vi "Display Hours Minutes Seconds.vi"() -> ()   [LabVIEW 2012]
panel:
  out "Time to Match (Hours:Minutes:Seconds)":dbl format="%<%H:%M:%S>t"
  out "Time to Match (Seconds / Milliseconds)":dbl
  out "Time to Match":i32
  out "No of Interations":i32
  out "Current Number":i32
  in  "Number to Match":i32=500000 min=0 max=1000000 step=1 format="%.0g"
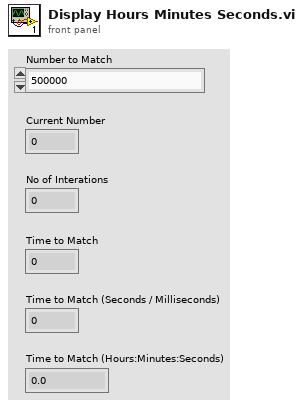
[diagram p1: front panel]
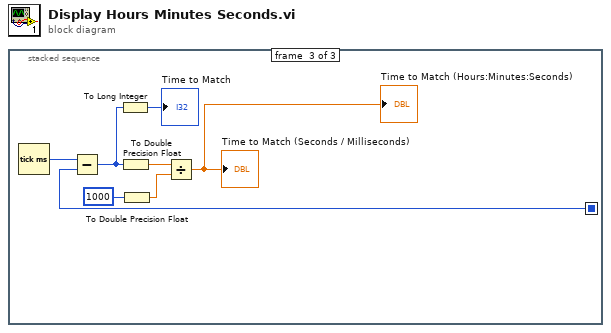
[diagram p0: block diagram]
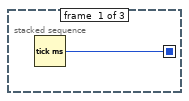
[diagram p2: hidden frame]
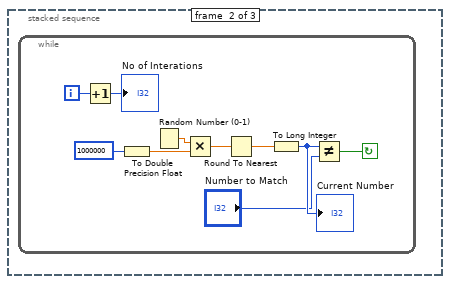
[diagram p3: hidden frame]
diagram:
  n1 = stacked-sequence {
    seq-local: [w1 _ _] -> [_ _ w18]
    frame #0 {
      n2 = Tick Count (ms)() -> (millisecond timer value=w1:u32)
    }
    frame #1 {
      n3 = while {
        i -> [w5]
        stop <- w2 continue-if-true
        n4 = Increment(x=w5) -> (x+1=→"No of Interations":i32)
        n5 = To Double Precision Float(number=1000000) -> (double precision float=w9:dbl)
        n6 = Random Number (0-1)() -> (number: 0 to 1=w11:dbl)
        n7 = Multiply(x=w11, y=w9) -> (x*y=w8:dbl)
        n8 = Round To Nearest(number=w8) -> (nearest integer value=w7:dbl)
        n9 = To Long Integer(number=w7) -> (32bit integer=w4:i32)
        "Current Number" <- w4
        n10 = Not Equal?(x=w4, y="Number to Match") -> (x != y?=w2:bool)
      }
    }
    frame #2 {
      n11 = Tick Count (ms)() -> (millisecond timer value=w19:u32)
      n12 = Subtract(x=w19, y=w18) -> (x-y=w14:u32)
      n13 = To Long Integer(number=w14) -> (32bit integer=→"Time to Match":i32)
      n14 = To Double Precision Float(number=w14) -> (double precision float=w13:dbl)
      n15 = To Double Precision Float(number=1000) -> (double precision float=w15:dbl)
      n16 = Divide(x=w13, y=w15) -> (x/y=→"Time to Match (Seconds / Milliseconds)" →"Time to Match (Hours:Minutes:Seconds)":dbl)
    }
  }
